vi "DWE Error Notifier.vi"(8 "Tab Control 3":refnum<vi>, 9 "Tab num":i32, 10 "Tab Control 2":T1(tab), 11 "Errors 1":T2) -> (2 "element":refnum<vi>)   [LabVIEW 2014]
uses:
  TypeDefs/DWE Errors.ctl
panel:
  out "Error":bool
  out "element 2":refnum<vi>
  in  "OK color":u32(colorbox)=12369084
  in  "y":bool
  out "error out":errorcluster
  in  "error in (no error)":errorcluster
  in  "Error color":u32(colorbox)=16726826
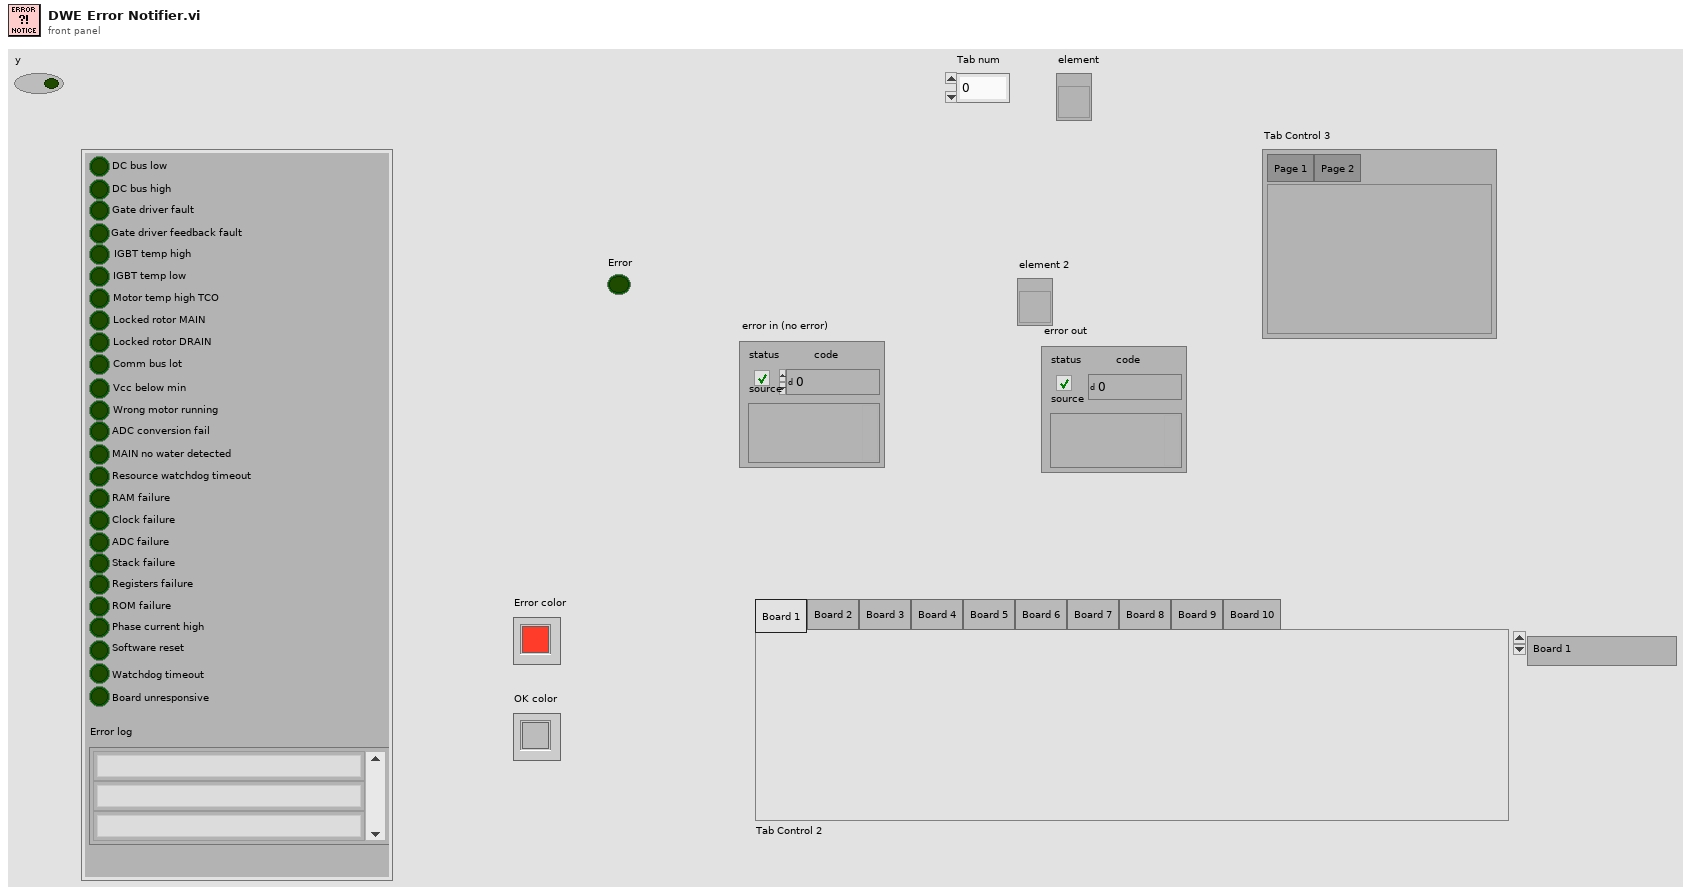
[diagram p1: front panel]
types:
  T1 = enum32{"Board 1", "Board 2", "Board 3", "Board 4", "Board 5", "Board 6", "Board 7", "Board 8", "Board 9", "Board 10"}
  T2 = typedef "DWE Errors.ctl" = cluster{"DC bus low":bool, "DC bus high":bool, "Gate driver fault":bool, "Gate driver feedback fault":bool, "IGBT temp high":bool, "IGBT temp low":bool, "Motor temp high TCO":bool, "Locked rotor MAIN":bool, "Locked rotor DRAIN":bool, "Comm bus lot":bool, "Vcc below min":bool, "Wrong motor running":bool, "ADC conversion fail":bool, "MAIN no water detected":bool, "Resource watchdog timeout":bool, "RAM failure":bool, "Clock failure":bool, "ADC failure":bool, "Stack failure":bool, "Registers failure":bool, "ROM failure":bool, "Phase current high":bool, "Software reset":bool, "Watchdog timeout":bool, "Error log":string[], "Board unresponsive":bool}
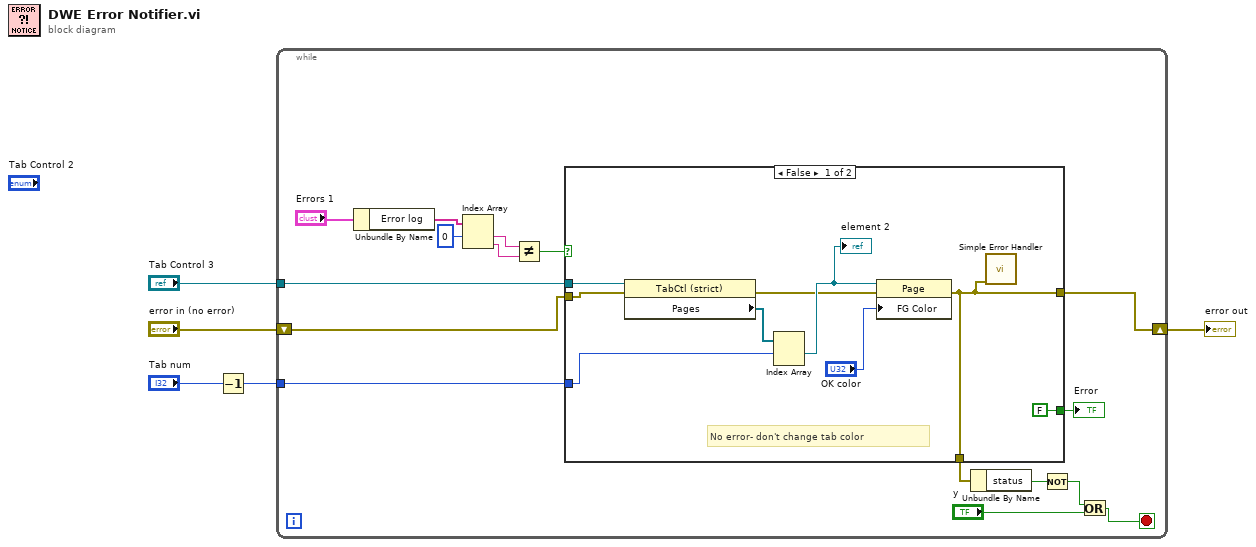
[diagram p0: block diagram]
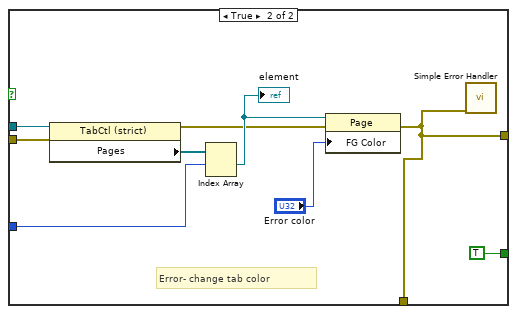
[diagram p2: hidden frame]
diagram:
  n1 = Decrement(x="Tab num") -> (x-1=w1:i32)
  n2 = while {
    tunnel: w1 -> [w16]
    shift-right: [w12] -> w4
    shift-left: "error in (no error)" -> [w8]
    tunnel: "Tab Control 3" -> [w9]
    stop <- w13 stop-if-true
    n3 = Unbundle By Name("Errors 1") -> ("Error log"=w20:string[])
    n4 = Index Array(array=w20, index #1=0 ("index")) -> (element #1=w18:string, element #2=w10:string)  [unwired: 1 in]
    n5 = Not Equal?(x=w18, y=w10) -> (x != y?=w17:bool)
    n6 = case shown="False" w17 {
      tunnel: w16 -> [w24 w38]
      tunnel: [w23 w36] -> w15
      tunnel: [w23 w36] -> w12
      tunnel: w9 -> [w25 w35]
      tunnel: w8 -> [w26 w34]
      tunnel: [FALSE TRUE] -> w6
      frame False {
        # "No error- don't change tab color"
        n7 = property class="TabCtl (strict)"(reference=w25, error in=w26) -> (error out=w27:errorcluster, "Pages"=w28:refnum<vi>[])  [unwired: 1 out]
        n8 = Index Array(array=w28, index #1=w24) -> (element #1=w29:refnum<vi>)  [unwired: 1 in, 1 out]
        "element 2" <- w29
        n9 = property class="Page"(reference=w29, error in=w27, "FG Color"="OK color") -> (error out=w23:errorcluster)  [unwired: 1 out]
        n10 = call <vilib>:"Simple Error Handler.vi"("error in (no error)"=w23) -> ()  [unwired: 4 in, 5 out]
      }
      frame True {
        # "Error- change tab color"
        n11 = property class="TabCtl (strict)"(reference=w35, error in=w34) -> (error out=w32:errorcluster, "Pages"=w33:refnum<vi>[])  [unwired: 1 out]
        n12 = Index Array(array=w33, index #1=w38) -> (element #1=w37:refnum<vi>)  [unwired: 1 in, 1 out]
        "element" <- w37
        n13 = property class="Page"(reference=w37, error in=w32, "FG Color"="Error color") -> (error out=w36:errorcluster)  [unwired: 1 out]
        n14 = call <vilib>:"Simple Error Handler.vi"("error in (no error)"=w36) -> ()  [unwired: 4 in, 5 out]
      }
    }
    "Error" <- w6
    n15 = Unbundle By Name(w15) -> ("status"=w11:bool)
    n16 = Not(x=w11) -> (.not. x?=w7:bool)
    n17 = Or(x=w7, y="y") -> (x .or. y?=w13:bool)
  }
  "error out" <- w4
